vi "create dictionary test.vi"() -> ()   [LabVIEW 2013, in "tag bus tests.lvlib"]
uses:
  tag bus tests.lvlib
  dictionary/data bus dictionary.lvclass
panel:
  in  "count":i32=5000
  out "lookup error":bool
  out "create error":errorcluster
  out "time":dbl
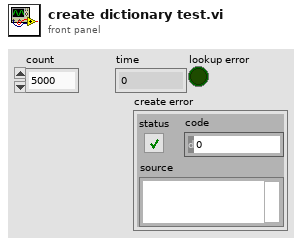
[diagram p1: front panel]
types:
  T1 = typedef "data bus tag description.lvclass/Data Type.ctl" = enum16{"Double", "I64", "Boolean", "Array of Double", "Array of I64", "Variant"}
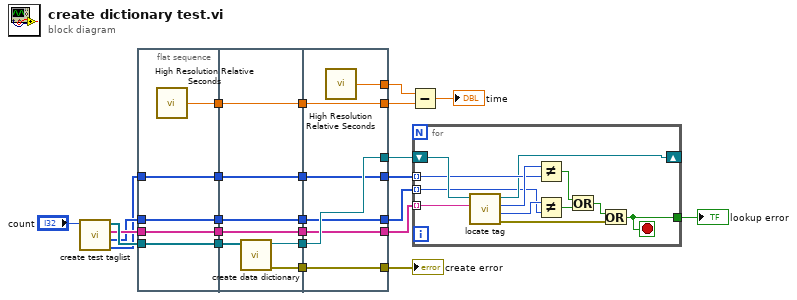
[diagram p0: block diagram]
diagram:
  n1 = call "create test taglist.vi"("count"="count") -> ("indices"=w8:i32[], "types"=w15:T1[], "names/metadata"=w18:string[], "tags"=w19:refnum<class "data bus tag description.lvclass">[])  [unwired: 7 in]
  n2 = flat-sequence {
    tunnel: [w30] -> w24
    tunnel: [w29] -> w20
    tunnel: w19 -> [w29]
    tunnel: w18 -> [w28]
    tunnel: [w28] -> w17
    tunnel: [w27] -> w16
    tunnel: w15 -> [w27]
    tunnel: [w26] -> w9
    tunnel: w8 -> [w26]
    tunnel: w24 -> [w37]
    tunnel: [w37] -> w23
    tunnel: w20 -> [w36]
    tunnel: w17 -> [w33]
    tunnel: w16 -> [w32]
    tunnel: [w35] -> w14
    tunnel: [w34] -> w13
    tunnel: [w33] -> w12
    tunnel: [w32] -> w11
    tunnel: [w31] -> w10
    tunnel: w9 -> [w31]
    tunnel: [w44] -> w25
    tunnel: w23 -> [w43]
    tunnel: [w43] -> w22
    tunnel: [w42] -> w7
    tunnel: w14 -> [w42]
    tunnel: [w41] -> w6
    tunnel: w13 -> [w41]
    tunnel: [w40] -> w5
    tunnel: w12 -> [w40]
    tunnel: [w39] -> w4
    tunnel: w11 -> [w39]
    tunnel: [w38] -> w3
    tunnel: w10 -> [w38]
    frame #0 {
      n3 = call <vilib>:"High Resolution Relative Seconds.vi"() -> ("relative seconds"=w30:dbl)
    }
    frame #1 {
      n4 = call "create data dictionary.vi"("system tags"=w36) -> ("error out"=w35:errorcluster, "data dictionary"=w34:refnum<class "data bus dictionary.lvclass">)  [unwired: 9 in]
    }
    frame #2 {
      n5 = call <vilib>:"High Resolution Relative Seconds.vi"() -> ("relative seconds"=w44:dbl)
    }
  }
  n6 = Subtract(x=w25, y=w22) -> (x-y=→"time":dbl)
  n7 = for {
    shift-right: [w50] -> _
    shift-left: w6 -> [w56]
    tunnel: w5 -> [w55] mode=indexing
    tunnel: w4 -> [w46] mode=indexing
    tunnel: w3 -> [w51] mode=indexing
    tunnel: [w49] -> w2
    stop <- w49 stop-if-true
    n8 = call "locate tag.vi"("name"=w55, "data dictionary in"=w56) -> ("error out"=w54:errorcluster, "data type"=w47:T1, "index"=w52:i32, "data dictionary out"=w50:refnum<class "data bus dictionary.lvclass">)  [unwired: 6 in]
    n9 = Not Equal?(x=w52, y=w51) -> (x != y?=w53:bool)
    n10 = Not Equal?(x=w47, y=w46) -> (x != y?=w45:bool)
    n11 = Or(x=w53, y=w45) -> (x .or. y?=w48:bool)
    n12 = Or(x=w48, y=w54) -> (x .or. y?=w49:bool)
  }
  "lookup error" <- w2
  "create error" <- w7
